vi "searcharray.vi"(1 "Search character":dbl, 2 "Array 2":dbl[](array[numeric])) -> (0 "Array":i16[](array[numeric]))   [LabVIEW 2014]
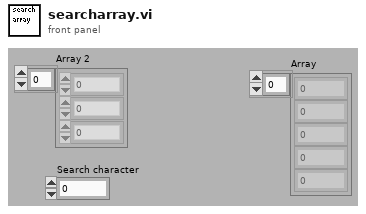
[diagram p1: front panel]
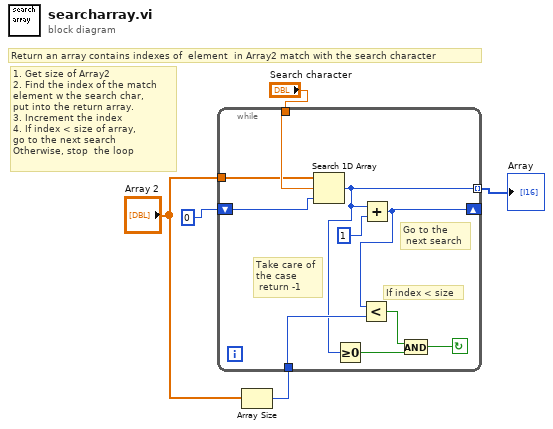
[diagram p0: block diagram]
diagram:
  # "1. Get size of Array2\n2. Find the index of the match \nelement w the search char,\nput into the return array.\n3. Increment the index\n4. If index < size of array,\ngo to the next search\nOtherwise, stop  the loop"
  # "Return an array contains indexes of  element  in Array2 match with the search character"
  n1 = Array Size(array="Array 2") -> (size(s)=w5:i32)
  n2 = while {
    tunnel: "Search character" -> [w15]
    tunnel: [w12] -> w4 mode=indexing
    shift-right: [w7] -> _
    shift-left: 0 -> [w6]
    tunnel: w5 -> [w13]
    tunnel: "Array 2" -> [w8]
    stop <- w9 continue-if-true
    # "If index < size"
    # "Take care of\nthe case\n return -1"
    # "Go to the\n next search"
    n3 = Search 1D Array(1D array=w8, element=w15, start index (0)=w6) -> (index of element=w12:i32)
    n4 = Greater Or Equal To 0?(x=w12) -> (x >= 0?=w11:bool)
    n5 = Add(x=w12, y=1) -> (x+y=w7:i32)
    n6 = Less?(x=w7, y=w13) -> (x < y?=w10:bool)
    n7 = And(x=w10, y=w11) -> (x .and. y?=w9:bool)
  }
  "Array" <- w4
